vi "Init Hosts List.vi"(8 "error in":errorcluster) -> (0 "error out":errorcluster)   [LabVIEW 2021, in "RT Interpreter.lvlib"]
uses:
  RT Interpreter.lvlib
  Connected Hosts List Action--enum.ctl
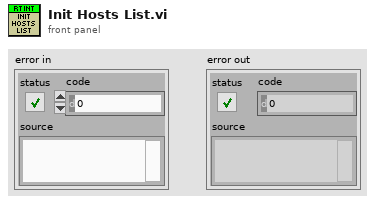
[diagram p1: front panel]
types:
  T1 = typedef "RT Interpreter.lvlib/Connected Hosts List Action--enum.ctl" = enum16{"Init", "Add Instance", "Remove Instance", "List Instances"}
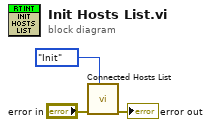
[diagram p0: block diagram]
diagram:
  n1 = call "Connected Hosts List.vi"("Action"=Connected_Hosts_List_Action--enum."Init", "error in"="error in") -> ("error out"=→"error out":errorcluster)  [unwired: 7 in, 2 out]
